vi "Load Built-in Error Codes.vi"(8 "error in (no error)":errorcluster) -> (0 "error out":errorcluster, 3 "error codes files content":T3(array[cluster]))   [LabVIEW 2017, in "Error File Management.lvlib"]
uses:
  Error File Management.lvlib
  Error List/Error Code File Properties.ctl
  Controls/NI Error.ctl
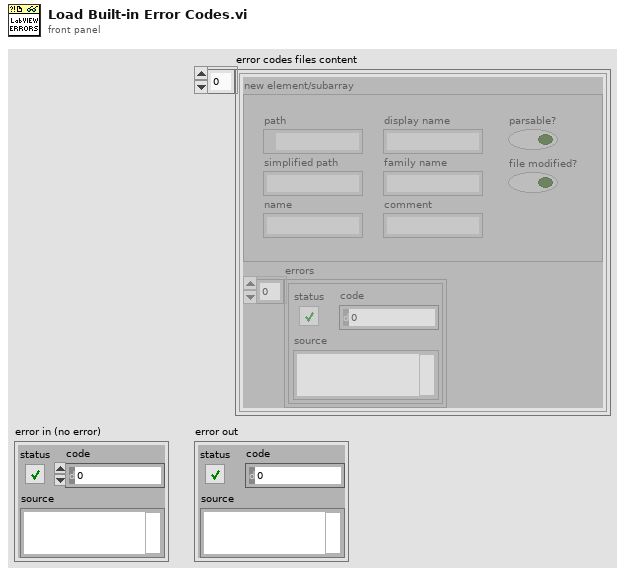
[diagram p1: front panel]
types:
  T1 = typedef "Error Code File Properties.ctl" = cluster{"path":path, "simplified path":string, "name":string, "display name":string, "family name":string, "comment":string, "parsable?":bool, "file modified?":bool}
  T2 = typedef "Error File Management.lvlib/NI Error.ctl" = errorcluster
  T3 = cluster{"new element/subarray":T1, "errors":T2[]}[]
  T4 = typedef "Error File Management.lvlib/NI Family.ctl" = cluster{"family name":string, "display name":string}
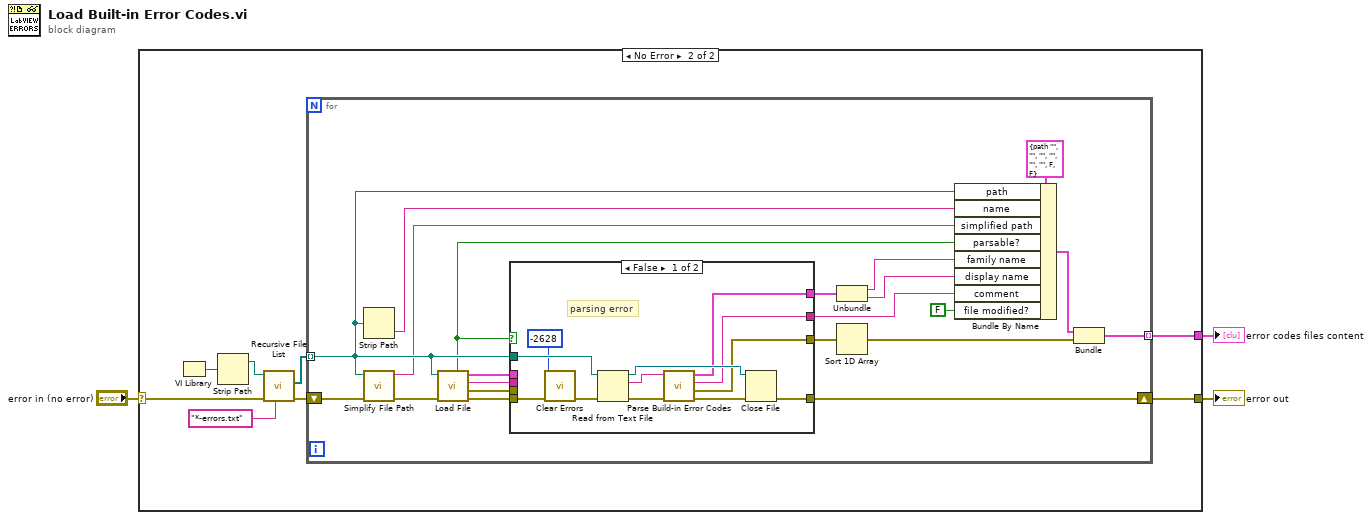
[diagram p0: block diagram]
diagram:
  n1 = case shown="No Error" "error in (no error)" {
    selector: "error in (no error)" -> [w4 w6]
    tunnel: [w4 w7] -> w2
    tunnel: [_ w5] -> w1
    frame Error {
    }
    frame No Error {
      n2 = VI Library() -> (path=w11:path)
      n3 = Strip Path(path=w11) -> (stripped path=w12:path)  [unwired: 1 out]
      n4 = call <vilib>:"Recursive File List.vi"("pattern"="*-errors.txt", "error in (no error)"=w6, "Folder Path"=w12) -> ("error out"=w8:errorcluster, "All Files in Dir"=w9:path[])  [unwired: 4 in, 3 out]
      n5 = for {
        tunnel: w9 -> [w33] mode=indexing
        shift-right: [w31] -> w7
        shift-left: w8 -> [w24]
        tunnel: [w13] -> w5 mode=indexing
        n6 = Strip Path(path=w33) -> (name=w22:string)  [unwired: 1 out]
        n7 = call "Simplify File Path.vi"("error in (no error)"=w24, "full path"=w33) -> ("error out"=w23:errorcluster, "simplified path"=w21:string)  [unwired: 8 in]
        n8 = call "Load File.vi"("error in (no error)"=w23, "error codes file"=w33) -> ("error out"=w30:errorcluster, "errors"=w29:T2[], "comment"=w28:string, "family"=w27:T4, "parsable?"=w32:bool)  [unwired: 5 in]
        n9 = case shown="False" w32 {
          tunnel: [w38 w49] -> w26
          tunnel: [w41 w48] -> w31
          tunnel: w33 -> [w40 _]
          tunnel: w30 -> [w39 w48]
          tunnel: w29 -> [_ w49]
          tunnel: w28 -> [_ w47]
          tunnel: w27 -> [_ w46]
          tunnel: [w37 w47] -> w17
          tunnel: [w36 w46] -> w20
          frame False {
            # "parsing error"
            n10 = call <vilib>:"Clear Errors.vi"("error in (no error)"=w39, "specific error code to clear (0: all)"=-2628) -> ("error out"=w35:errorcluster)  [unwired: 4 in, 1 out]
            n11 = Read from Text File(file (use dialog)=w40, error in=w35) -> (refnum out=w44:refnum<file>, text=w45:string, error out=w43:errorcluster)  [unwired: 2 in, 1 out]
            n12 = call "Parse Build-in Error Codes.vi"("error in (no error)"=w43, "errors file content"=w45) -> ("error out"=w42:errorcluster, "errors"=w38:T2[], "comment"=w37:string, "family"=w36:T4)  [unwired: 6 in]
            n13 = Close File(refnum=w44, error in=w42) -> (error out=w41:errorcluster)  [unwired: 1 out]
          }
          frame True {
          }
        }
        n14 = Unbundle(w20) -> ("family name"=w19:string, "display name"=w18:string)
        n15 = Sort 1D Array(array=w26) -> (sorted array=w14:T2[])
        n16 = Bundle By Name(cluster=T1 {"path"=path "", "simplified path"="", "name"="", "display name"="", "family name"="", "comment"="", "parsable?"=FALSE, "file modified?"=FALSE} ("new element/subarray"), "path"=w33, "name"=w22, "simplified path"=w21, "parsable?"=w32, "family name"=w19, "display name"=w18, "comment"=w17, "file modified?"=FALSE) -> (w15:T1)
        n17 = Bundle("new element/subarray"=w15, w14) -> (w13:cluster{"new element/subarray":T1, T2[]})  [unwired: 1 in]
      }
    }
  }
  "error out" <- w2
  "error codes files content" <- w1
